vi "Task4.vi"() -> ()   [LabVIEW 2017]
panel:
  out "Waveform Chart":u32(graph)
  in  "stop":bool
  out "Numeric":dbl
  in  "Button":bool[](array[boolean])
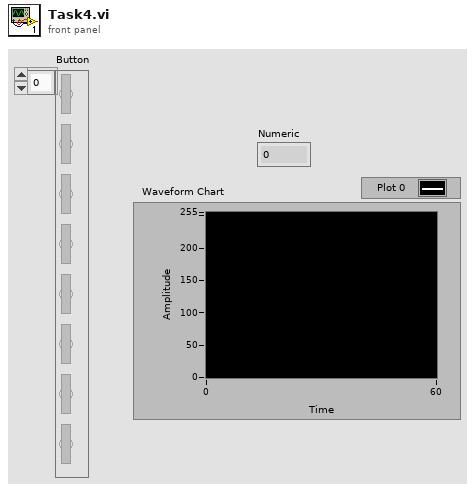
[diagram p1: front panel]
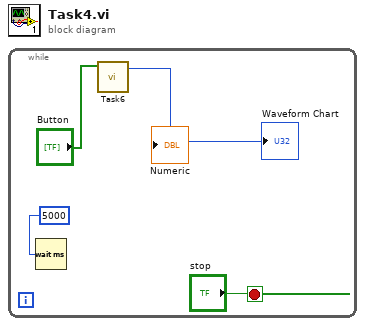
[diagram p0: block diagram]
diagram:
  n1 = while {
    stop <- "stop" stop-if-true
    n2 = Wait (ms)(milliseconds to wait=5000) -> ()  [unwired: 1 out]
    n3 = call "Task6.vi"("Button"="Button") -> ("Numeric"=→"Numeric" →"Waveform Chart":u32)  [unwired: 10 in]
  }
